vi "Serial Commands Engineering Tool.vi"() -> ()   [LabVIEW 2012]
uses:
  Type Defs/Final Output.ctl
panel:
  out "Cal Data":T1={"Time"="20:36:08", "Consecutive good readings"=4, "Total readings"=-1, "A/D counts Sensor 1"=3314.919, "A/D counts Sensor 2"=3314.935, "Diff current/previous Sensor 1"=-0.155, "Diff current/previous Sensor 2"=-0.099}
  out "Data Read":T2={"Date"="03/14/13", "Time"="51:50:28", "CO2- ppm"=1354, "Last Ctrl Word"=400000, "O2-1 ppm"=208212, "O2-2 ppm"=208179, "Temp MB"=23.6, "Temp Sensor Module"=25.29, "Press mB"=838.96}
  in  "Other Outputs":cluster{"Alarm":bool, "Heater":bool}
  in  "Final Output":T3
  in  "Start O2 Calibration 5-10 Minutes":bool
  in  "Check Firmware":bool
  in  "Read RT Clock":bool
  out "Current error":errorcluster
  in  "Set RT Clock":bool
  in  "error in":errorcluster
  in  "CAT On/Off":bool
  in  "Date string":string="02/17/13,02/117/13,21:27:00,1"
  out "Version":string="Ver. 0.1, Feb 10 2013, 23:27:07\r\n"
  out "RT Clock":string="03/14/13,12/01/13,22:00:39,5\r\n"
  in  "Com Parms":T4={"VISA resource name"="COM3", "baud rate"=38400, "data bits"=8, "parity"=0, "stop bits"=10, "flow control"=0} {"flow control" items=["None"=0, "XON/XOFF"=1, "RTS/CTS"=2, "DTR/DSR"=4]; "stop bits" items=["1.0"=10, "1.5"=15, "2.0"=20]; "parity" items=["None", "Odd", "Even", "Mark", "Space"]; "data bits" min=5 max=8 step=1}
  in  "stop":bool
  # "Set prior to running"
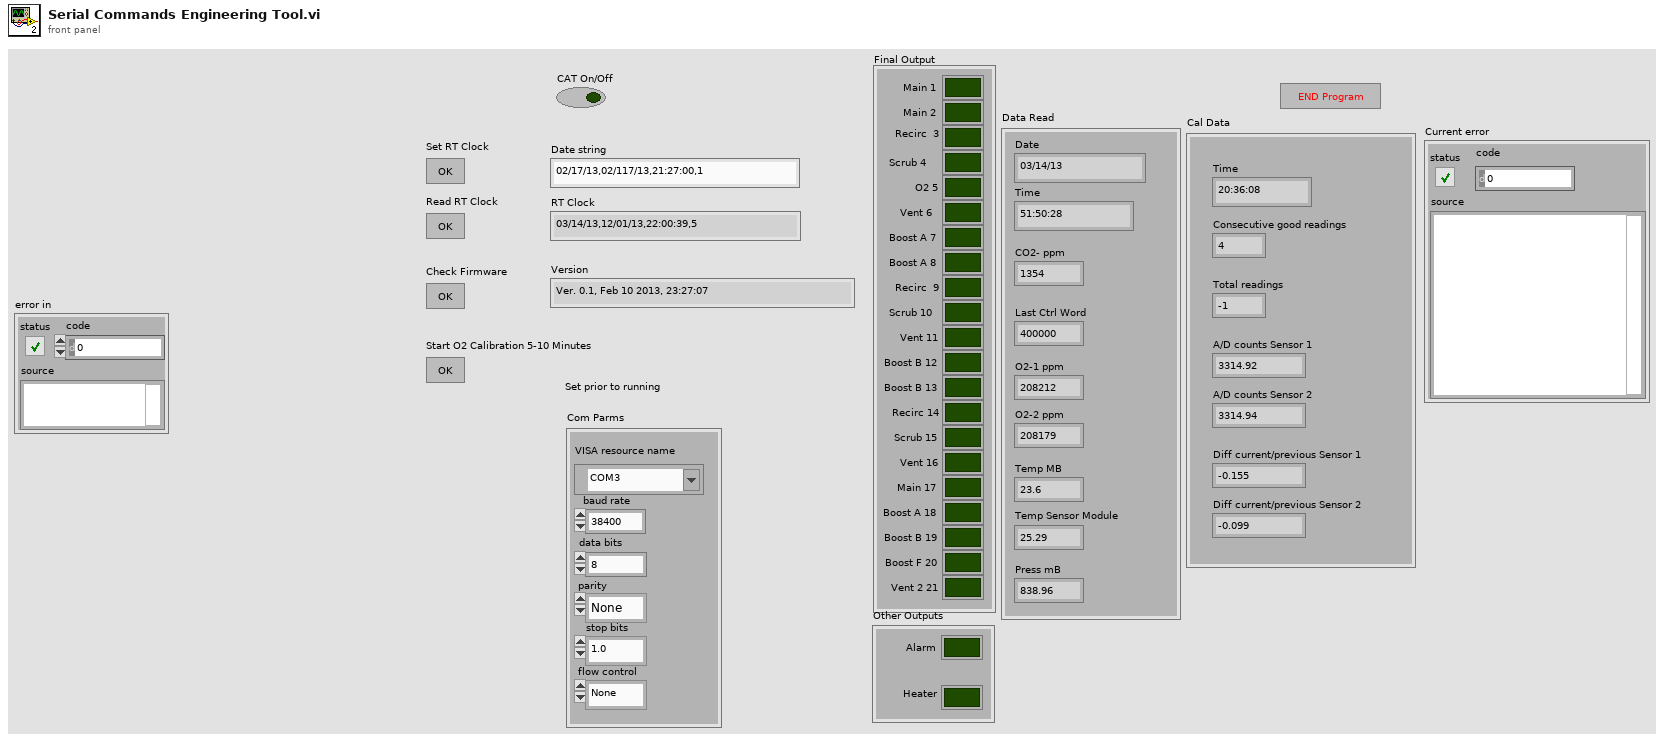
[diagram p1: front panel]
types:
  T1 = cluster{"Time":string, "Consecutive good readings":i32, "Total readings":i32, "A/D counts Sensor 1":sgl, "A/D counts Sensor 2":sgl, "Diff current/previous Sensor 1":sgl, "Diff current/previous Sensor 2":sgl}
  T2 = cluster{"Date":string, "Time":string, "CO2- ppm":u32, "Last Ctrl Word":u32, "O2-1 ppm":u32, "O2-2 ppm":u32, "Temp MB":sgl, "Temp Sensor Module":sgl, "Press mB":sgl}
  T3 = typedef "Final Output.ctl" = cluster{"Main 1":bool, "Main 2":bool, "Recirc  3":bool, "Scrub 4":bool, "O2 5":bool, "Vent 6":bool, "Boost A 7":bool, "Boost A 8":bool, "Recirc  9":bool, "Scrub 10":bool, "Vent 11":bool, "Boost B 12":bool, "Boost B 13":bool, "Recirc 14":bool, "Scrub 15":bool, "Vent 16":bool, "Main 17":bool, "Boost A 18":bool, "Boost B 19":bool, "Boost F 20":bool, "Vent 2 21":bool}
  T4 = cluster{"VISA resource name":refnum<visa-resource-name>, "baud rate":u32, "data bits":u16, "parity":u16, "stop bits":u16, "flow control":u16}
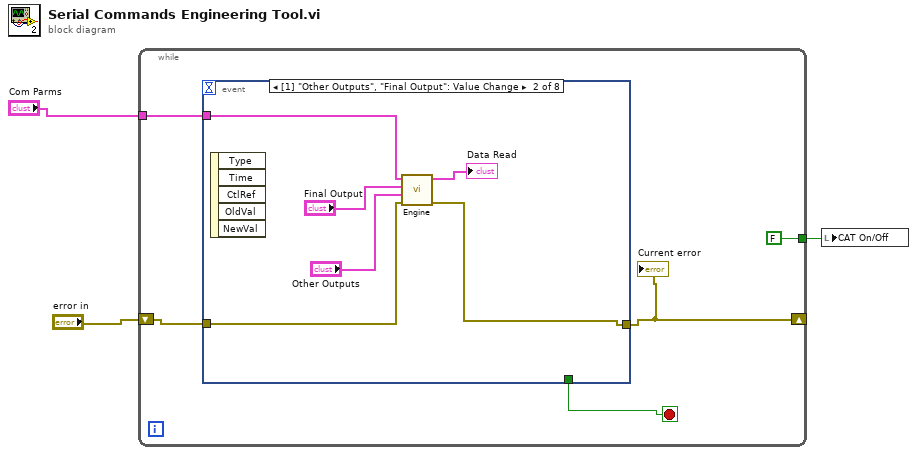
[diagram p0: block diagram]
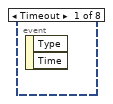
[diagram p2: hidden frame]
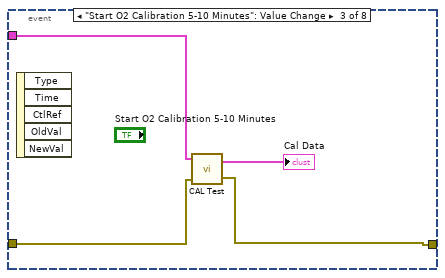
[diagram p3: hidden frame]
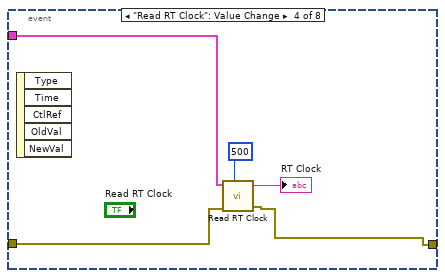
[diagram p4: hidden frame]
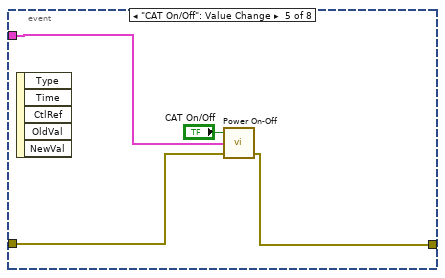
[diagram p5: hidden frame]
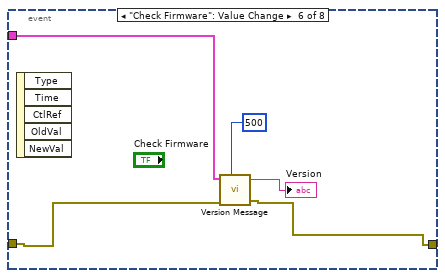
[diagram p6: hidden frame]
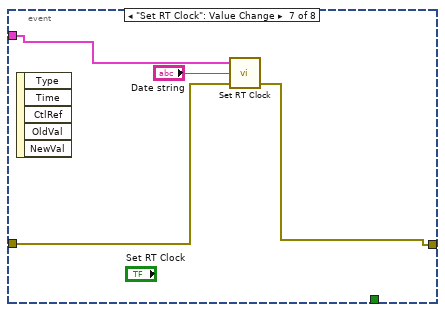
[diagram p7: hidden frame]
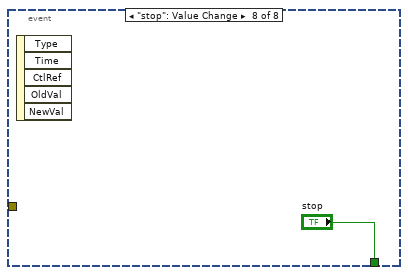
[diagram p8: hidden frame]
diagram:
  n1 = while {
    tunnel: "Com Parms" -> [w8]
    shift-right: [w6] -> _
    shift-left: "error in" -> [w7]
    tunnel: [FALSE ("CAT On/Off")] -> w1
    stop <- w5 stop-if-true
    n2 = event shown="[1] \"Other Outputs\", \"Final Output\": Value Change" {
      selector: _ -> [_ _ _ _ _ _ _ _]
      dyn-events: _ -> [_ _ _ _ _ _ _ _]
      timeout: _ -> [_ _ _ _ _ _ _ _]
      tunnel: w8 -> [_ w9 w16 w20 w24 w29 w33 _]
      tunnel: w7 -> [_ w11 w18 w22 w26 w31 w35 _]
      tunnel: [_ w10 w17 w21 w25 w30 w34 _] -> w6
      tunnel: [_ _ _ _ _ _ _ "stop"] -> w5
      event Timeout {
        n3 = event-data() -> ()  [unwired: 1 in, 2 out]
      }
      event "Other Outputs": Value Change {
        n4 = event-data() -> ()  [unwired: 1 in, 5 out]
        n5 = call "Engine.vi"("error in"=w11, "Other Outputs"="Other Outputs", "Final Output Controls"="Final Output", "Com Parms"=w9) -> ("error out"=w10:errorcluster, "Data Read"=→"Data Read":T2)  [unwired: 3 in]
      }
      event "Start O2 Calibration 5-10 Minutes": Value Change {
        n6 = event-data() -> ()  [unwired: 1 in, 5 out]
        n7 = call "CAL Test.vi"("error in (no error)"=w18, "Com Parms"=w16) -> ("error out"=w17:errorcluster, "Cal Data"=→"Cal Data":T1)  [unwired: 2 in]
      }
      event "Read RT Clock": Value Change {
        n8 = event-data() -> ()  [unwired: 1 in, 5 out]
        n9 = call "Read RT Clock.vi"("Com Parms"=w20, "delay before read (ms)"=u32 500, "error in"=w22) -> ("read string"=→"RT Clock":string, "error out"=w21:errorcluster)  [unwired: 4 in]
      }
      event "CAT On/Off": Value Change {
        n10 = event-data() -> ()  [unwired: 1 in, 5 out]
        n11 = call "Power On-Off.vi"("error in"=w26, "Com Parms"=w24, "On/Off"="CAT On/Off") -> ("error out"=w25:errorcluster)  [unwired: 2 in]
      }
      event "Check Firmware": Value Change {
        n12 = event-data() -> ()  [unwired: 1 in, 5 out]
        n13 = call "Version Message.vi"("Com Parms"=w29, "delay before read (ms)"=u32 500, "error in"=w31) -> ("read string"=→"Version":string, "error out"=w30:errorcluster)  [unwired: 4 in]
      }
      event "Set RT Clock": Value Change {
        n14 = event-data() -> ()  [unwired: 1 in, 5 out]
        n15 = call "Set RT Clock.vi"("error in"=w35, "Date string"="Date string", "Com Parms"=w33) -> ("error out"=w34:errorcluster)  [unwired: 2 in]
      }
      event "stop": Value Change {
        n16 = event-data() -> ()  [unwired: 1 in, 5 out]
      }
    }
    "Current error" <- w6
  }
  n17 = local write "CAT On/Off"(w1) -> ()
